vi "Close ProviderVI.vi"(8 "error in (no error)":errorcluster, 11 "VI in":refnum<vi>) -> (0 "error out":errorcluster)   [LabVIEW 2019, in "LabVIEW-VIProviderShell.lvlib" / "VIProviderShellHelper.lvclass"]
uses:
  VIProviderShellHelper.lvclass
  50c25862-178f-4498-86b1-4e3779e48a1e.vi
  <vilib>/Utility/error.llb/Clear Errors.vi
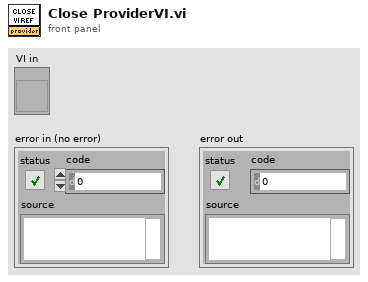
[diagram p1: front panel]
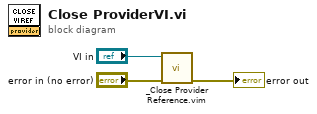
[diagram p0: block diagram]
diagram:
  n1 = call "_Close Provider Reference.vim"("error in (no error)"="error in (no error)", "LVClassLibrary in"="VI in") -> ("error out"=→"error out":errorcluster)  [unwired: 9 in]
